vi "GradosCaF.vi"(1 "Temperatura gC":dbl) -> (0 "Temperatura gF":dbl)   [LabVIEW 2020]
doc: "Esta funcion convierte una temperatura de grados C a grados F"
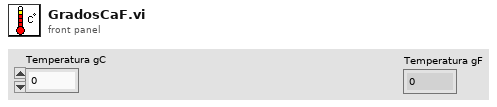
[diagram p1: front panel]
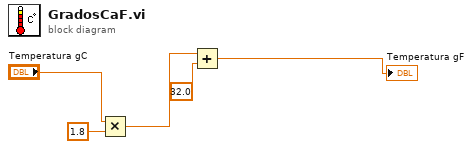
[diagram p0: block diagram]
diagram:
  n1 = Multiply(x="Temperatura gC", y=1.8) -> (x*y=w3:dbl)
  n2 = Add(x=w3, y=32.0) -> (x+y=→"Temperatura gF":dbl)
